vi "Generate CV command.vi"(8 "Error in":errorcluster, 11 "CV configuration":T1={"E begin (V)"=0.0, "E vertex 1 (V)"=0.0, "E vertex 2 (V)"=0.0, "Cycles"=1, "Scan rate (V/s)"=0.01, "E step (V)"=0.01} {"E step (V)" min=0.01 max=0.25; "Scan rate (V/s)" min=0.01 max=10.0; "Cycles" min=1; "E vertex 2 (V)" min=-3.3 max=3.3; "E vertex 1 (V)" min=-3.3 max=3.3; "E begin (V)" min=-3.3 max=3.3}) -> (0 "Error out":errorcluster, 3 "Paquet command":u8[](array[numeric]) format="%02x")   [LabVIEW 2021]
uses:
  Typedefs/CV configuration.ctl
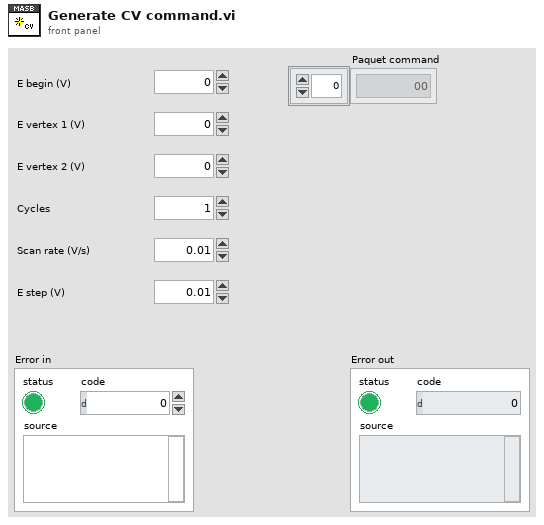
[diagram p1: front panel]
types:
  T1 = typedef "CV configuration.ctl" = cluster{"E begin (V)":dbl, "E vertex 1 (V)":dbl, "E vertex 2 (V)":dbl, "Cycles":u8, "Scan rate (V/s)":dbl, "E step (V)":dbl}
  T2 = enum16{"big-endian, network order", "native, host order", "little-endian"}
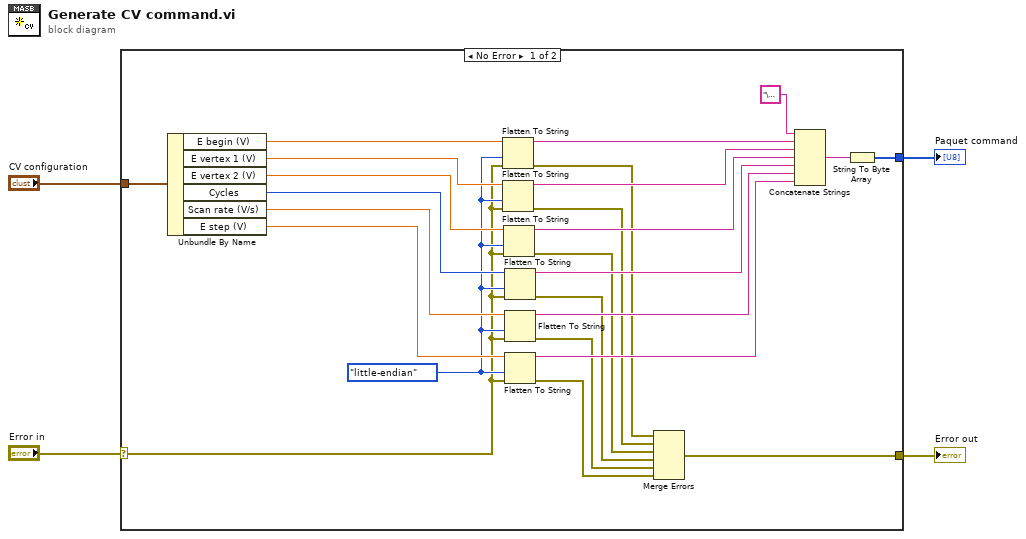
[diagram p0: block diagram]
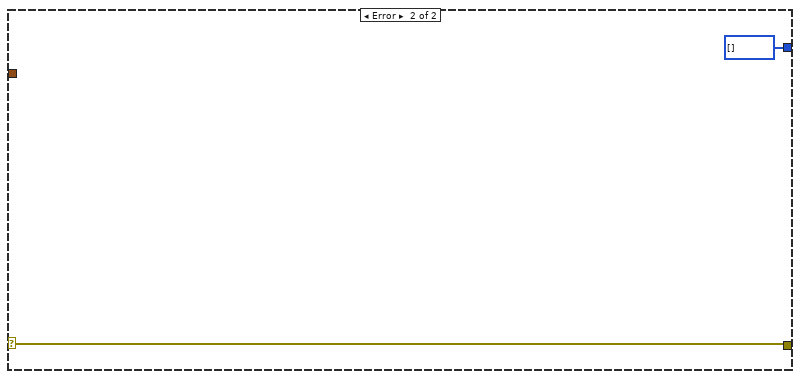
[diagram p2: hidden frame]
diagram:
  n1 = case shown="No Error" "Error in" {
    selector: "Error in" -> [w5 w31]
    tunnel: [w8 u8[] [] ("unsigned byte array")] -> w4
    tunnel: [w7 w31] -> w3
    tunnel: "CV configuration" -> [w6 _]
    frame No Error {
      w9 = T2."little-endian" ("byte order (0:big-endian, network order)")
      n2 = Unbundle By Name(w6) -> ("E begin (V)"=w25:dbl, "E vertex 1 (V)"=w24:dbl, "E vertex 2 (V)"=w23:dbl, "Cycles"=w22:u8, "Scan rate (V/s)"=w21:dbl, "E step (V)"=w20:dbl)
      n3 = Flatten To String(anything=w25, byte order (0:big-endian, network order)=w9, error in (no error)=w5) -> (data string=w29:string, error out=w15:errorcluster)  [unwired: 1 in, 1 out]
      n4 = Flatten To String(anything=w24, byte order (0:big-endian, network order)=w9, error in (no error)=w5) -> (data string=w28:string, error out=w14:errorcluster)  [unwired: 1 in, 1 out]
      n5 = Flatten To String(anything=w23, byte order (0:big-endian, network order)=w9, error in (no error)=w5) -> (data string=w19:string, error out=w13:errorcluster)  [unwired: 1 in, 1 out]
      n6 = Flatten To String(anything=w22, byte order (0:big-endian, network order)=w9, error in (no error)=w5) -> (data string=w18:string, error out=w12:errorcluster)  [unwired: 1 in, 1 out]
      n7 = Flatten To String(anything=w21, byte order (0:big-endian, network order)=w9, error in (no error)=w5) -> (data string=w17:string, error out=w11:errorcluster)  [unwired: 1 in, 1 out]
      n8 = Flatten To String(anything=w20, byte order (0:big-endian, network order)=w9, error in (no error)=w5) -> (data string=w16:string, error out=w10:errorcluster)  [unwired: 1 in, 1 out]
      n9 = Merge Errors(w15, w14, w13, w12, w11, w10) -> (w7:errorcluster)
      n10 = Concatenate Strings("\u0001" ("string"), w29, w28, w19, w18, w17, w16) -> (w26:string)
      n11 = String To Byte Array(string=w26) -> (unsigned byte array=w8:u8[])
    }
    frame Error {
    }
  }
  "Paquet command" <- w4
  "Error out" <- w3
